vi "Init Pneumatics Pack.vi"() -> ()   [LabVIEW 2018]
uses:
  <vilib>/Rock Robotics/WPI/Solenoid/WPI_SolenoidChannel.ctl
  <vilib>/Rock Robotics/WPI/Solenoid/WPI_SolenoidValue.ctl
  <vilib>/Rock Robotics/WPI/Solenoid/WPI_SolenoidOpenDouble.vi
  <vilib>/Rock Robotics/WPI/Solenoid/WPI_SolenoidSetEnum.vi
  <vilib>/Rock Robotics/WPI/Utilities/WPI_GetSetVariantRefNum.vi
panel:
  in  "Intake Retract Channel":T1=enum."Solenoid 6"
  in  "Intake Extend Channel":T1=enum."Solenoid 7"
  in  "Claw Retract Channel":T1
  in  "Claw Extend Channel":T1=enum."Solenoid 1"
  in  "Kicker Close Channel":T1=enum."Solenoid 5"
  in  "Kicker Open Channel":T1=enum."Solenoid 4"
  in  "Gripper Close Channel":T1=enum."Solenoid 3"
  in  "Gripper Open Channel":T1=enum."Solenoid 2"
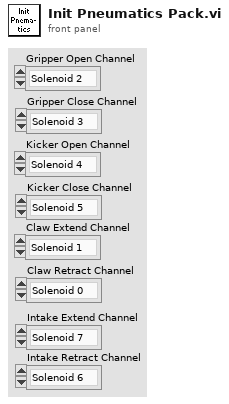
[diagram p1: front panel]
types:
  T1 = typedef "WPI_SolenoidChannel.ctl" = enum8{"Solenoid 0", "Solenoid 1", "Solenoid 2", "Solenoid 3", "Solenoid 4", "Solenoid 5", "Solenoid 6", "Solenoid 7", "Invalid"}
  T2 = typedef "WPI_SolenoidValue.ctl" = enum16{"Off", "On", "Forward", "Reverse"}
  T3 = typedef "WPI_CompressorDevRef.ctl" = cluster{"DevStatus":errorcluster, "Pneumatics Control Module":u8}
  T4 = typedef "WPI_SolenoidDevRef.ctl" = cluster{"DevStatus":errorcluster, "Pneumatics Control Module":u8, "Forward Solenoid Channel":T1, "Reverse Solenoid Channel":T1}
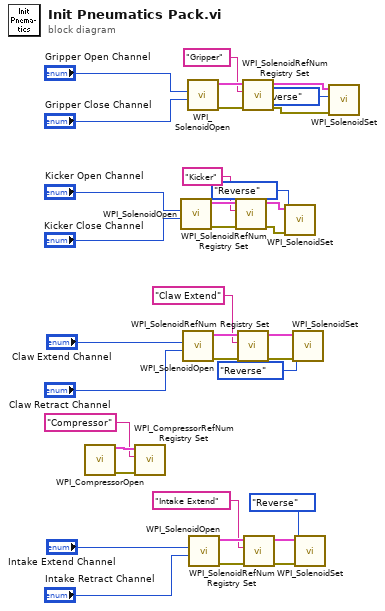
[diagram p0: block diagram]
diagram:
  n1 = call <vilib>:"WPI_CompressorOpen.vi"() -> ("CompressorDevRef"=w28:T3, "error out"=w29:errorcluster)  [unwired: 14 in]
  n2 = call <vilib>:"WPI_CompressorRefNum Registry Set.vi"("error in (no error)"=w29, "refnum name"="Compressor", "CompressorDevRef"=w28) -> ()  [unwired: 7 in, 2 out]
  n3 = call-poly <vilib>:"WPI_SolenoidOpen.vi"("Reverse Solenoid Channel"="Kicker Close Channel", "Forward Solenoid Channel"="Kicker Open Channel") -> ("error out"=w22:errorcluster, "SolenoidDevRef"=w23:T4)  [unwired: 8 in]
  n4 = call-poly <vilib>:"WPI_SolenoidOpen.vi"("Reverse Solenoid Channel"="Claw Retract Channel", "Forward Solenoid Channel"="Claw Extend Channel") -> ("error out"=w27:errorcluster, "SolenoidDevRef"=w26:T4)  [unwired: 8 in]
  n5 = call-poly <vilib>:"WPI_SolenoidOpen.vi"("Reverse Solenoid Channel"="Gripper Close Channel", "Forward Solenoid Channel"="Gripper Open Channel") -> ("error out"=w24:errorcluster, "SolenoidDevRef"=w25:T4)  [unwired: 8 in]
  n6 = call-poly <vilib>:"WPI_SolenoidOpen.vi"("Reverse Solenoid Channel"="Intake Retract Channel", "Forward Solenoid Channel"="Intake Extend Channel") -> ("error out"=w17:errorcluster, "SolenoidDevRef"=w16:T4)  [unwired: 8 in]
  n7 = call <vilib>:"WPI_SolenoidRefNum Registry Set.vi"("error in (no error)"=w22, "refnum name"="Kicker", "SolenoidDevRef"=w23) -> ("error out"=w5:errorcluster, "SolenoidDevRef"=w6:T4)  [unwired: 7 in]
  n8 = call <vilib>:"WPI_SolenoidRefNum Registry Set.vi"("error in (no error)"=w27, "refnum name"="Claw Extend", "SolenoidDevRef"=w26) -> ("error out"=w8:errorcluster, "SolenoidDevRef"=w9:T4)  [unwired: 7 in]
  n9 = call <vilib>:"WPI_SolenoidRefNum Registry Set.vi"("error in (no error)"=w24, "refnum name"="Gripper", "SolenoidDevRef"=w25) -> ("error out"=w2:errorcluster, "SolenoidDevRef"=w3:T4)  [unwired: 7 in]
  n10 = call <vilib>:"WPI_SolenoidRefNum Registry Set.vi"("error in (no error)"=w17, "refnum name"="Intake Extend", "SolenoidDevRef"=w16) -> ("error out"=w12:errorcluster, "SolenoidDevRef"=w11:T4)  [unwired: 7 in]
  n11 = call-poly <vilib>:"WPI_SolenoidSet.vi"("error in (no error)"=w5, "Value"=WPI_SolenoidValue."Reverse", "SolenoidDevRef"=w6) -> ()  [unwired: 7 in, 2 out]
  n12 = call-poly <vilib>:"WPI_SolenoidSet.vi"("error in (no error)"=w8, "Value"=WPI_SolenoidValue."Reverse", "SolenoidDevRef"=w9) -> ()  [unwired: 7 in, 2 out]
  n13 = call-poly <vilib>:"WPI_SolenoidSet.vi"("error in (no error)"=w12, "Value"=WPI_SolenoidValue."Reverse", "SolenoidDevRef"=w11) -> ()  [unwired: 7 in, 2 out]
  n14 = call-poly <vilib>:"WPI_SolenoidSet.vi"("error in (no error)"=w2, "Value"=WPI_SolenoidValue."Reverse", "SolenoidDevRef"=w3) -> ()  [unwired: 7 in, 2 out]
